vi "Get Results.vi"(8 "error in (no error)":errorcluster, 11 "Abstract Results Msg in":refnum<class "Abstract Results Msg.lvclass">) -> (0 "error out":errorcluster, 2 "Results":variant, 3 "Abstract Results Msg out":refnum<class "Abstract Results Msg.lvclass">)   [LabVIEW 2013, in "Hot And Cold Source Unit Model.lvlib" / "Abstract Results Msg.lvclass"]
uses:
  Abstract Results Msg.lvclass
  Abstract Results Msg.lvclass/Abstract Results Msg.ctl
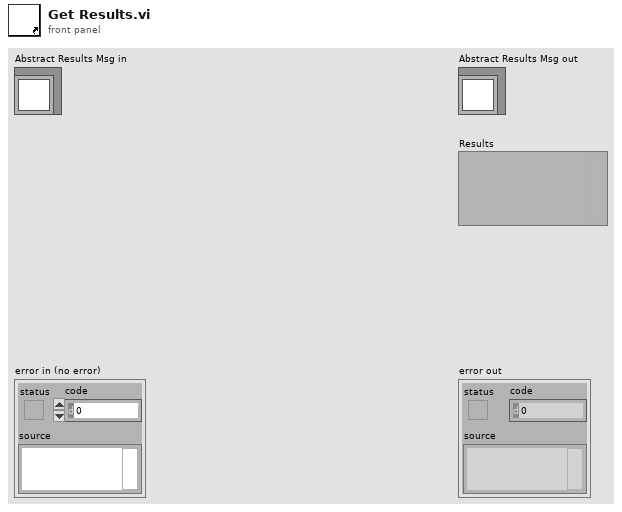
[diagram p1: front panel]
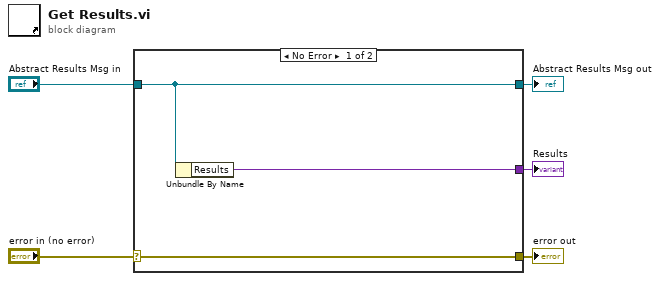
[diagram p0: block diagram]
diagram:
  n1 = case shown="No Error" "error in (no error)" {
    selector: "error in (no error)" -> [w8 w9]
    tunnel: [w8 w9] -> w4
    tunnel: [w7 w10] -> w2
    tunnel: "Abstract Results Msg in" -> [w7 w10]
    tunnel: [w6 _] -> w1
    frame No Error {
      n2 = Unbundle By Name(w7) -> ("Results"=w6:variant)
    }
    frame Error {
    }
  }
  "error out" <- w4
  "Abstract Results Msg out" <- w2
  "Results" <- w1
